vi "ex_HMSToSeconds.vi"(2 "seconds":i32, 3 "minutes":i32, 4 "hours":i32) -> (0 "seconds":i32)   [LabVIEW 2017]
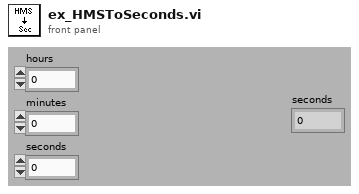
[diagram p1: front panel]
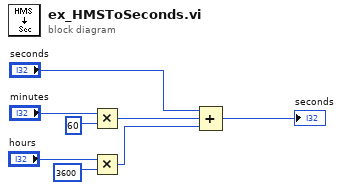
[diagram p0: block diagram]
diagram:
  n1 = Multiply(x="minutes", y=60 ("seconds")) -> (x*y=w4:i32)
  n2 = Multiply(x="hours", y=3600 ("seconds")) -> (x*y=w3:i32)
  n3 = Compound Arithmetic op=ADD("seconds", w4, w3) -> (→"seconds":i32)
